vi "Z_Stage_Movement.vi"(9 "Z Input":dbl) -> (1 "Current Z Position":sgl)   [LabVIEW 2013]
panel:
  out "Original Z Position":sgl
  in  "Z Stage Serial":i32
  in  "Z Stage Motor":refnum<k7>(container)
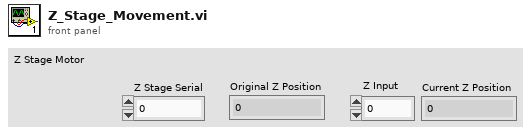
[diagram p1: front panel]
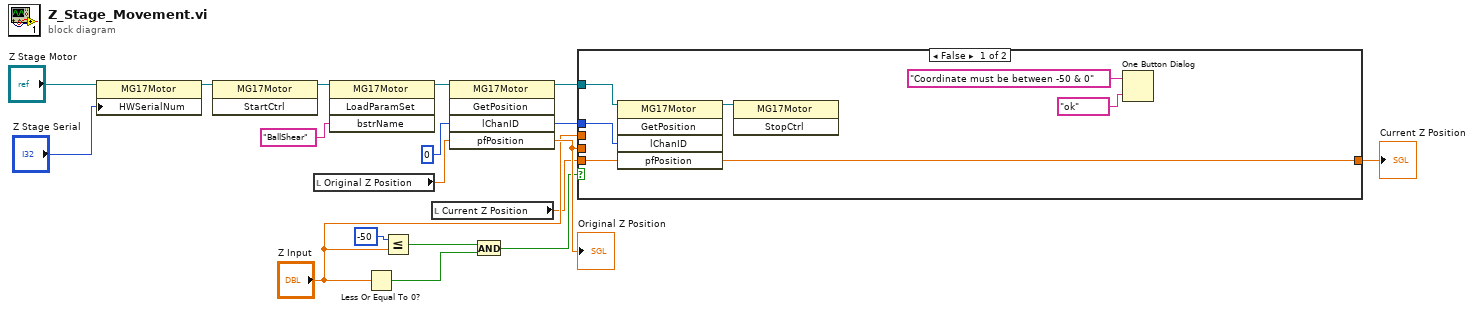
[diagram p0: block diagram]
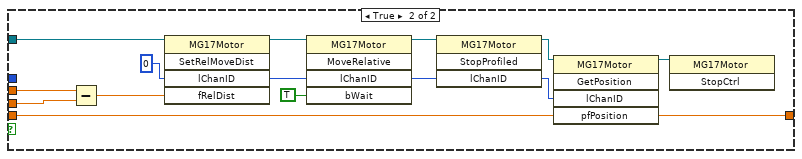
[diagram p2: hidden frame]
diagram:
  n1 = property class="MG17Motor"(reference="Z Stage Motor", "HWSerialNum"="Z Stage Serial") -> (reference out=w16:refnum<k7>)  [unwired: 1 in, 1 out]
  n2 = invoke class="MG17Motor" method="StartCtrl"(reference=w16) -> (reference out=w4:refnum<k7>)  [unwired: 2 in, 2 out]
  n3 = local read "Original Z Position"() -> (w14:sgl)
  n4 = invoke class="MG17Motor" method="LoadParamSet"(reference=w4, "bstrName"="BallShear") -> (reference out=w5:refnum<k7>)  [unwired: 2 in, 3 out]
  n5 = Less Or Equal To 0?(x="Z Input") -> (x <= 0?=w7:bool)
  n6 = Less Or Equal?(x=-50, y="Z Input") -> (x <= y?=w9:bool)
  n7 = local read "Current Z Position"() -> (w3:sgl)
  n8 = invoke class="MG17Motor" method="GetPosition"(reference=w5, "lChanID"=0, "pfPosition"=w14) -> (reference out=w11:refnum<k7>, "lChanID"=w1:i32, "pfPosition"=w13:sgl)  [unwired: 2 in, 2 out]
  "Original Z Position" <- w13
  n9 = And(x=w9, y=w7) -> (x .and. y?=w12:bool)
  n10 = case shown="False" w12 {
    tunnel: "Z Input" -> [_ w31]
    tunnel: w13 -> [_ w32]
    tunnel: w11 -> [w25 w33]
    tunnel: [w21 w28] -> w2
    tunnel: w3 -> [w22 w27]
    tunnel: w1 -> [w19 _]
    frame False {
      n11 = invoke class="MG17Motor" method="GetPosition"(reference=w25, "lChanID"=w19, "pfPosition"=w22) -> (reference out=w20:refnum<k7>, "pfPosition"=w21:sgl)  [unwired: 2 in, 3 out]
      n12 = invoke class="MG17Motor" method="StopCtrl"(reference=w20) -> ()  [unwired: 2 in, 3 out]
      n13 = One Button Dialog(message="Coordinate must be between -50 & 0", button name ("OK")="ok") -> ()  [unwired: 1 out]
    }
    frame True {
      n14 = Subtract(x=w31, y=w32) -> (x-y=w34:dbl)
      n15 = invoke class="MG17Motor" method="SetRelMoveDist"(reference=w33, "lChanID"=0, "fRelDist"=w34) -> (reference out=w37:refnum<k7>, "lChanID"=w38:i32)  [unwired: 2 in, 3 out]
      n16 = invoke class="MG17Motor" method="MoveRelative"(reference=w37, "lChanID"=w38, "bWait"=TRUE) -> (reference out=w39:refnum<k7>, "lChanID"=w40:i32)  [unwired: 2 in, 3 out]
      n17 = invoke class="MG17Motor" method="StopProfiled"(reference=w39, "lChanID"=w40) -> (reference out=w26:refnum<k7>, "lChanID"=w30:i32)  [unwired: 2 in, 2 out]
      n18 = invoke class="MG17Motor" method="GetPosition"(reference=w26, "lChanID"=w30, "pfPosition"=w27) -> (reference out=w29:refnum<k7>, "pfPosition"=w28:sgl)  [unwired: 2 in, 3 out]
      n19 = invoke class="MG17Motor" method="StopCtrl"(reference=w29) -> ()  [unwired: 2 in, 3 out]
    }
  }
  "Current Z Position" <- w2
